vi "例4-6.vi"() -> ()   [LabVIEW 2019]
panel:
  in  "停止":bool
  out "报警指示":bool
  in  "温度报警限值":dbl=75.0
  out "温度计":dbl(slide) scale=0.0..100.0
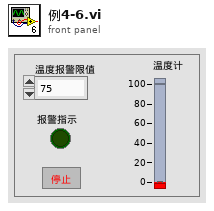
[diagram p1: front panel]
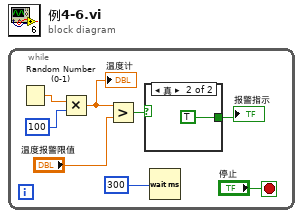
[diagram p0: block diagram]
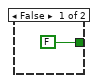
[diagram p2: hidden frame]
diagram:
  n1 = while {
    stop <- "停止" stop-if-true
    n2 = Random Number (0-1)() -> (number: 0 to 1=w8:dbl)
    n3 = Multiply(x=w8, y=100) -> (x*y=w4:dbl)
    "温度计" <- w4
    n4 = Greater?(x=w4, y="温度报警限值") -> (0:w6:bool)
    n5 = case shown="真" w6 {
      tunnel: [FALSE TRUE] -> w3
      frame False {
      }
      frame True {
      }
    }
    "报警指示" <- w3
    n6 = Wait (ms)(milliseconds to wait=300) -> ()  [unwired: 1 out]
  }
